vi "force_clamp.vi"(8 "error in (no error)":errorcluster, 9 "Boolean":bool, 10 "y":dbl, 11 "handle in":i32) -> (0 "error out":errorcluster)   [LabVIEW 2019]
uses:
  controller/SubVIs_nanostage/Madlib.dll
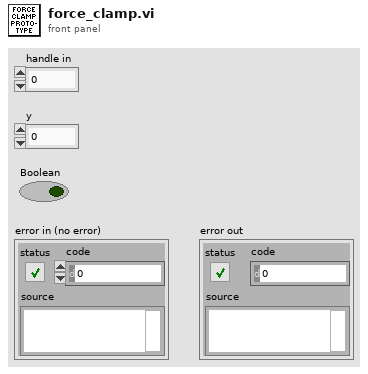
[diagram p1: front panel]
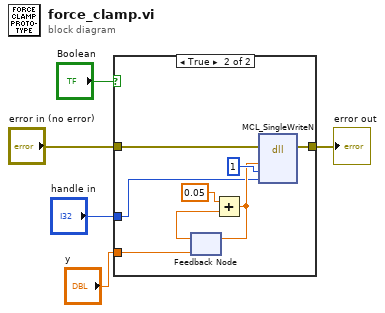
[diagram p0: block diagram]
diagram:
  n1 = case shown="True" "Boolean" {
    tunnel: "handle in" -> [_ w10]
    tunnel: "error in (no error)" -> [w6 w9]
    tunnel: [w6 w8] -> w4
    tunnel: "y" -> [_ w7]
    frame False {
    }
    frame True {
      n2 = feedback #1(w7) -> (w11:dbl)
      n3 = Add(x=0.05, y=w11) -> (x+y=w12:dbl)
      n4 = feedback-in #1(w12) -> ()
      n5 = dll-call lib="C:/Users/admin/Desktop/controller/SubVIs_nanostage/MADLib.dll" fn="MCL_SingleWriteN"(error in=w9, "position"=w12, "axis"=u32 1, "handle"=w10) -> (error out=w8:errorcluster)  [unwired: 6 in, 1 out]
    }
  }
  "error out" <- w4
